vi "New INI Key for DIR.vi"(9 "Default Path":path=path "C:/Incoming", 10 "INI key (in)":string="Scan Rats Directory", 11 "INI section (in)":string="File Paths") -> (2 "output cluster":T1)   [LabVIEW 2010]
uses:
  <vilib>/Utility/sysdir.llb/System Directory Type.ctl
  <vilib>/Utility/config.llb/Read Key (Path).vi
  <vilib>/Utility/config.llb/NI_LVConfig.lvlib
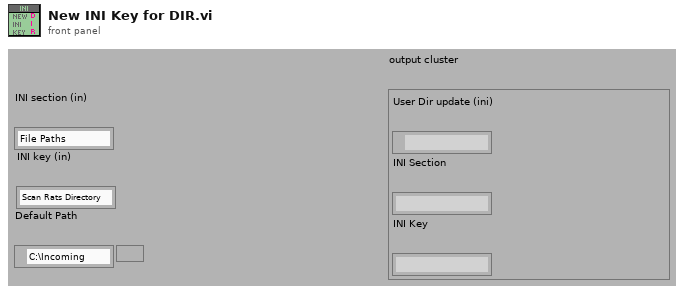
[diagram p1: front panel]
types:
  T1 = cluster{"User Dir update (ini)":path, "INI Section":string, "INI Key":string}
  T2 = cluster{"local Var of File Path":path, "INI section":string, "INI key":string}
  T3 = typedef "System Directory Type.ctl" = i32
  T4 = typedef "NI_LVConfig.lvlib/Config Data RefNum.ctl" = refnum<k1>
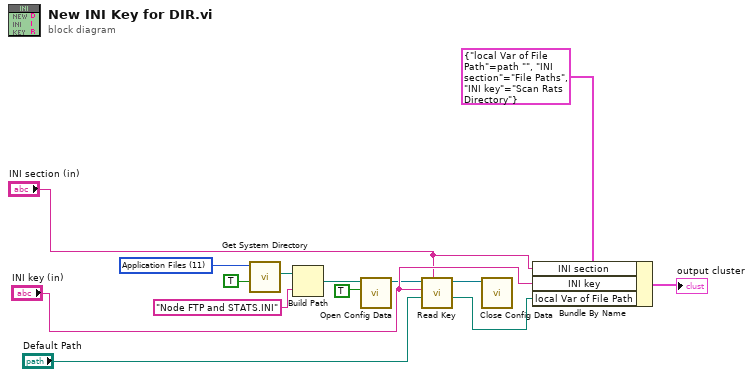
[diagram p0: block diagram]
diagram:
  w3 = T3 11 items=["User Home"=0, "User Desktop"=1, "User Documents"=2, "User Application Data"=3, "User Preferences"=4, "User Temporary"=5, "Public Documents"=6, "Public Application Data"=7, "Public Preferences"=8, "Public Cache"=13, "System Core Libraries"=9, "System Installed Libraries"=10, "Application Files"=11, "Boot Volume Root"=12] ("system directory type")
  n1 = call <vilib>:"Get System Directory.vi"("create directory if not found? (F)"=TRUE, "system directory type"=w3) -> ("system directory"=w4:path)  [unwired: 9 in]
  n2 = Build Path(base path=w4, name or relative path="Node FTP and STATS.INI") -> (appended path=w6:path)
  n3 = call <vilib>:"Open Config Data.vi"("create file if necessary (T)"=TRUE, "configuration file path"=w6) -> ("refnum"=w7:T4)  [unwired: 7 in, 2 out]
  n4 = call-poly <vilib>:"Read Key.vi"("section"="INI section (in)", "default value"="Default Path", "key"="INI key (in)", "refnum"=w7) -> ("value"=w13:path, "refnum out"=w9:T4)  [unwired: 4 in, 2 out]
  n5 = call <vilib>:"Close Config Data.vi"("refnum"=w9) -> ()  [unwired: 9 in, 2 out]
  n6 = Bundle By Name(cluster=T2 {"local Var of File Path"=path "", "INI section"="File Paths", "INI key"="Scan Rats Directory"} ("Cluster"), "INI section"="INI section (in)", "INI key"="INI key (in)", "local Var of File Path"=w13) -> (→"output cluster":T2)
